vi "Image_Crop_Fixed.vi"(8 "Particle Measurements":dbl[][](array[numeric])=[[57.0, 126.0, 60.0, 134.0, 14.0], [248.0, 156.0, 341.0, 306.0, 6231.0], [31.0, 193.0, 32.0, 194.0, 1.0], [324.0, 201.0, 327.0, 209.0, 15.0], [350.0, 252.0, 359.0, 273.0, 108.0], [55.0, 573.0, 56.0, 576.0, 3.0]], 9 "Image  in":T1, 11 "Data":T2={"Pinch-valve"="Test Sample", "XLP 6000 Pump"="MRJ", "Camera1"="", "Camera2"="", "Img_Capt"=FALSE, "Actuator"=FALSE, "Pump"=FALSE, "Cam 1"=FALSE, "Cam 2"=FALSE, "Empty_Refill"=FALSE, "Crop"=FALSE, "Light intensity"=0, "Exposure Time"=0.0, "Sample Name"="", "Operator"="", "Calibration 1"=path "C:/Users/au540322/Desktop/IHS_Project/images/Debris/Debris_0/Debris_0_2019_06_01-23-32-49-686.PNG", "Calibration 2"=path "C:/Users/au540322/Desktop/IHS_Project/images/Debris/Debris_0/Debris_0_2019_06_01-23-32-49-686.PNG", "Framerate"=1, "Timeout Sample"=1, "Collection date"="", "Sample size threshold"=500, "Empty start"=500, "Command"="", "Station"="", "Species Name"="", "Other Notes"="", "Aperture"=enum."Item 3", "Image Process Queue Size"=100, "Image Save Queue Size"=0, "Overload threshold"=0, "Max Framerate"=0, "Rectangle 1"={"Left"=0, "Top"=0, "Right"=0, "Bottom"=0, "Rotation"=0.0}, "Rectangle 2"={"Left"=0, "Top"=100, "Right"=100, "Bottom"=0, "Rotation"=0.0}, "Detection Region %"=200.0, "Detect 1"=path "C:/Users/au540322/Desktop/IHS_Project/images/Debris/Debris_0/Debris_0_2019_06_01-23-32-49-686.PNG", "Detect 2"=path "C:/Users/au540322/Desktop/IHS_Project/images/Debris/Debris_0/Debris_0_2019_06_01-23-32-49-686.PNG", "Max large object threshold"=500, "Open(T)/Close(F)"=FALSE, "Img_Capt Begin"=FALSE, "Dispense Speed"=0, "Flush Size"=0, "Location"="", "Latitude"="", "Longitude"="", "Determiner"="", "Sex"="", "Camera1_Img"=refnum, "Camera2_Img"=refnum, "Img1_Orig_Disp"=refnum, "Img2_Orig_Disp"=refnum, "Img1_Orig_RGB"=refnum, "Img2_Orig_RGB"=refnum, "Blue_Plane_Extract"=refnum, "Subtracted_Plane"=refnum, "Img1_Binary"=refnum, "Img2_Binary"=refnum, "Crop_Mask"=refnum, "Img1_Save"=refnum, "Img2_Save"=refnum, "Img1_Cali_Full"=refnum, "Img2_Cali_Full"=refnum, "Img1_Cali_Detect"=refnum, "Img2_Cali_Detect"=refnum, "Cam 1 queue"=refnum, "Cam 2 queue"=refnum, "Cam 1 - save queue"=refnum, "Cam 2 - save queue"=refnum, "Overlay_Ring"=0, "SystemVersion"=0, "System Serial"="", "Legacy Cam Attributes"=FALSE, "Camera Orientation 1"="", "Camera Orientation 2"="", "Pixel to mm 1"=0.0, "Pixel to mm 2"=0.0} {"SystemVersion" items=["Standard", "XL"]; "Overlay_Ring" items=["Session Data", "Extended Setup", "Buffer", "Camera", "Dispenser", "Stats", "Connections"]; "Flush Size" min=1; "Dispense Speed" min=1; "Rectangle 2"."Rotation" format="%.2f"; "Rectangle 2"."Left" scale=0.0..1024.0; "Rectangle 2"."Right" scale=0.0..1024.0; "Rectangle 1"."Rotation" format="%.2f"; "Rectangle 1"."Left" scale=0.0..1024.0; "Rectangle 1"."Right" scale=0.0..1024.0; "Max Framerate" min=1; "Overload threshold" min=1; "Image Save Queue Size" min=1; "Image Process Queue Size" min=1; "Empty start" min=1; "Sample size threshold" min=1; "Framerate" min=1; "Light intensity" scale=0.0..100.0}) -> (0 "ROI descriptor":T5={"Global Rectangle"=[233, 141, 356, 321], "Contours"=[{"ID"=enum."External", "Type"=3, "Coordinates"=[233, 141, 356, 321]}]}, 2 "Object accept":bool=TRUE, 3 "Object":bool)   [LabVIEW 2022 SP3]
uses:
  controls/Data.ctl
  <vilib>/userdefined/High Color/IMAQdx.ctl
  <vilib>/vision/Image Controls.llb/IMAQ Image.ctl
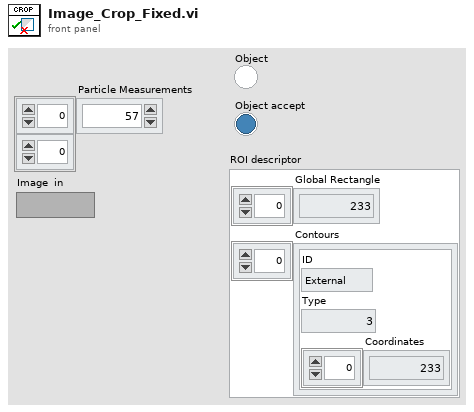
[diagram p1: front panel]
types:
  T1 = typedef "IMAQ Image.ctl" = refnum<image>
  T2 = typedef "Data.ctl" = cluster{"Pinch-valve":refnum<visa-resource-name>, "XLP 6000 Pump":refnum<visa-resource-name>, "Camera1":T3, "Camera2":T3, "Img_Capt":bool, "Actuator":bool, "Pump":bool, "Cam 1":bool, "Cam 2":bool, "Empty_Refill":bool, "Crop":bool, "Light intensity":i32, "Exposure Time":dbl, "Sample Name":string, "Operator":string, "Calibration 1":path, "Calibration 2":path, "Framerate":i32, "Timeout Sample":i32, "Collection date":string, "Sample size threshold":i32, "Empty start":u32, "Command":string, "Station":string, "Species Name":string, "Other Notes":string, "Aperture":enum32{"Item 0", "Item 1", "Item 2", "Item 3"}, "Image Process Queue Size":i32, "Image Save Queue Size":i32, "Overload threshold":i32, "Max Framerate":i32, "Rectangle 1":T4, "Rectangle 2":T4, "Detection Region %":dbl, "Detect 1":path, "Detect 2":path, "Max large object threshold":i32, "Open(T)/Close(F)":bool, "Img_Capt Begin":bool, "Dispense Speed":i32, "Flush Size":i32, "Location":string, "Latitude":string, "Longitude":string, "Determiner":string, "Sex":string, "Camera1_Img":T1, "Camera2_Img":T1, "Img1_Orig_Disp":T1, "Img2_Orig_Disp":T1, "Img1_Orig_RGB":T1, "Img2_Orig_RGB":T1, "Blue_Plane_Extract":T1, "Subtracted_Plane":T1, "Img1_Binary":T1, "Img2_Binary":T1, "Crop_Mask":T1, "Img1_Save":T1, "Img2_Save":T1, "Img1_Cali_Full":T1, "Img2_Cali_Full":T1, "Img1_Cali_Detect":T1, "Img2_Cali_Detect":T1, "Cam 1 queue":refnum<queue>, "Cam 2 queue":refnum<queue>, "Cam 1 - save queue":refnum<queue>, "Cam 2 - save queue":refnum<queue>, "Overlay_Ring":u16, "SystemVersion":u16, "System Serial":string, "Legacy Cam Attributes":bool, "Camera Orientation 1":string, "Camera Orientation 2":string, "Pixel to mm 1":dbl, "Pixel to mm 2":dbl}
  T3 = typedef "IMAQdx.ctl" = refnum<k21>
  T4 = typedef "IMAQ Rectangle" = cluster{"Left":i32, "Top":i32, "Right":i32, "Bottom":i32, "Rotation":dbl}
  T5 = cluster{"Global Rectangle":i32[], "Contours":cluster{"ID":enum32{"External", "Internal"}, "Type":u32, "Coordinates":i32[]}[]}
  T6 = cluster{"ID":enum32{"External", "Internal"}, "Type":u32, "Coordinates":i32[]}[]
  T7 = cluster{"ID":enum32{"External", "Internal"}, "Type":u32, "Coordinates":i32[]}
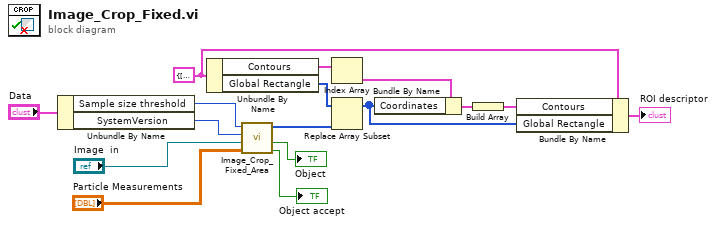
[diagram p0: block diagram]
diagram:
  w9 = T5 {"Global Rectangle"=[106, 29, 356, 265], "Contours"=[{"ID"=enum."External", "Type"=3, "Coordinates"=[106, 29, 356, 265]}]} ("Crop to object")
  n1 = Unbundle By Name("Data") -> ("Sample size threshold"=w7:i32, "SystemVersion"=w1:u16)
  n2 = Unbundle By Name(w9) -> ("Contours"=w15:T6, "Global Rectangle"=w16:i32[])
  n3 = call "Image_Crop_Fixed_Area.vi"("Particle Measurements in"="Particle Measurements", "Image  in"="Image  in", "SystemVersion"=w1, "Object size threshold"=w7) -> ("Object accept"=→"Object accept":bool, "Object"=→"Object":bool, "Crop coordinates array"=w8:i32[])  [unwired: 5 in]
  n4 = Index Array(array=w15) -> (element=w14:T7)  [unwired: 1 in]
  n5 = Replace Array Subset(array=w16, new element=w8) -> (w13:i32[])  [unwired: 1 in]
  n6 = Bundle By Name(cluster=w14, "Coordinates"=w13) -> (w12:T7)
  n7 = Build Array(w12) -> (w11:T6)
  n8 = Bundle By Name(cluster=w9, "Contours"=w11, "Global Rectangle"=w13) -> (→"ROI descriptor":T5)
